vi "Tick.vi"(8 "error in (no error)":errorcluster, 9 "Any elements read?":bool, 11 "ScopeBase in":refnum<class "ScopeBase.lvclass">) -> (0 "error out":errorcluster, 3 "ScopeBase out":refnum<class "ScopeBase.lvclass">)   [LabVIEW 2013, in "ScopeBase.lvclass"]
uses:
  ScopeBase.lvclass
  ScopeBase.lvclass/ScopeBase.ctl
  controls/ScopeMode.ctl
  Utilities/Ticker/Ticker.lvclass
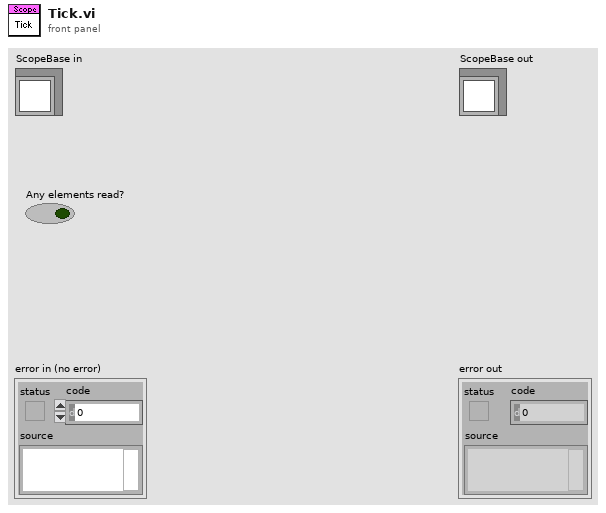
[diagram p1: front panel]
types:
  T1 = typedef "ScopeMode.ctl" = enum16{"Stopped", "Single", "Running", "Continuous"}
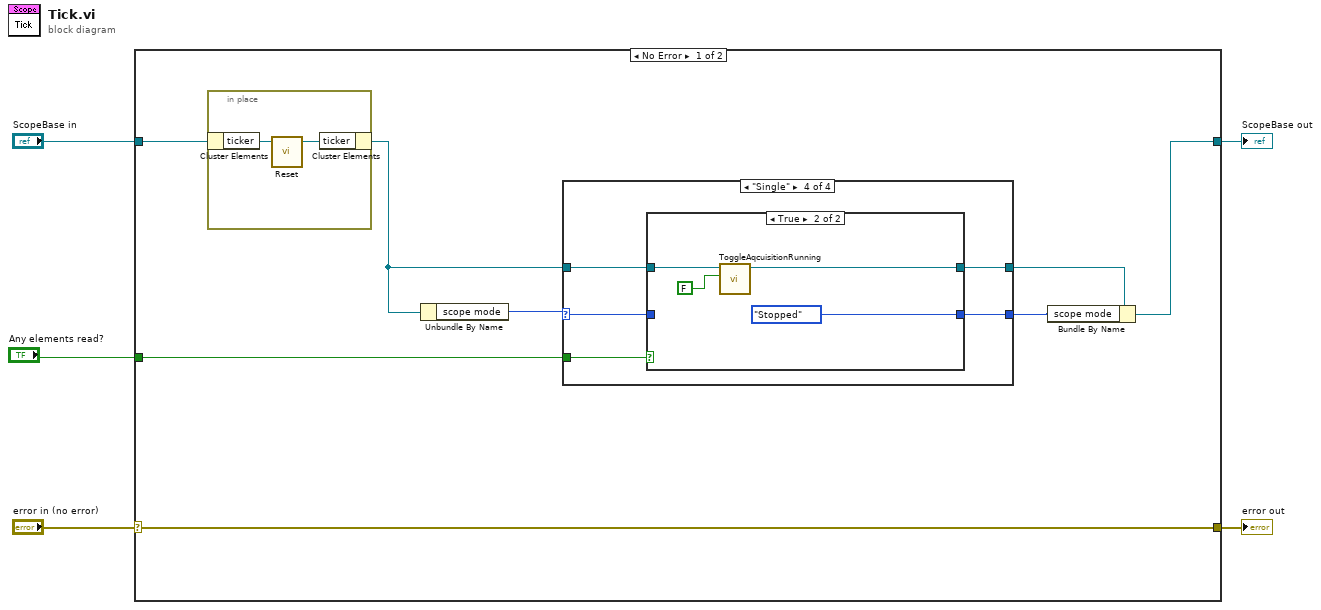
[diagram p0: block diagram]
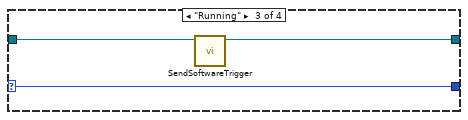
[diagram p4: hidden frame]
diagram:
  n1 = case shown="No Error" "error in (no error)" {
    selector: "error in (no error)" -> [w12 w34]
    tunnel: [w12 w34] -> w4
    tunnel: [w6 w33] -> w2
    tunnel: "ScopeBase in" -> [w11 w33]
    tunnel: "Any elements read?" -> [w9 _]
    frame No Error {
      n2 = in-place {
        n3 = in-place-cluster #1(w11) -> ("ticker"=w32:refnum<class "Ticker.lvclass">)
        n4 = call "Reset.vi"("Ticker in"=w32) -> ("Ticker out"=w31:refnum<class "Ticker.lvclass">)  [unwired: 9 in, 1 out]
        n5 = in-place-cluster #1("ticker"=w31) -> ()  [unwired: 1 out]
      }
      n6 = Unbundle By Name(w11) -> ("scope mode"=w10:T1)
      n7 = case shown="\"Single\"" w10 {
        selector: w10 -> [w14 w16 w19 w20]
        tunnel: [w14 w16 w19 w24] -> w7
        tunnel: w11 -> [w13 w15 w17 w22]
        tunnel: [w13 w15 w18 w21] -> w8
        tunnel: w9 -> [_ _ _ w23]
        frame "Stopped" {
        }
        frame "Continuous" {
        }
        frame "Running" {
          n8 = call-dynamic "SendSoftwareTrigger.vi"("ScopeBase In"=w17) -> ("ScopeBase Out"=w18:refnum<class "ScopeBase.lvclass">)  [unwired: 9 in, 1 out]
        }
        frame "Single" {
          n9 = case shown="True" w23 {
            tunnel: [w25 ScopeMode."Stopped" ("scope mode")] -> w24
            tunnel: w22 -> [w26 w27]
            tunnel: [w26 w29] -> w21
            tunnel: w20 -> [w25 _]
            frame False {
            }
            frame True {
              n10 = call-dynamic "ToggleAqcuisitionRunning.vi"("Acquisition running"=FALSE, "ScopeBase In"=w27) -> ("ScopeBase Out"=w29:refnum<class "ScopeBase.lvclass">)  [unwired: 8 in, 1 out]
            }
          }
        }
      }
      n11 = Bundle By Name(cluster=w8, "scope mode"=w7) -> (w6:refnum<class "ScopeBase.lvclass">)
    }
    frame Error {
    }
  }
  "error out" <- w4
  "ScopeBase out" <- w2
